vi "channels_get.vi"(8 "error in (no error)":errorcluster, 11 "OSA300 in":refnum<class "OSA300.lvclass">) -> (0 "error out":errorcluster, 1 "channel properties":T1(array[cluster]), 2 "channels nr":i32, 3 "OSA300 out":refnum<class "OSA300.lvclass">)   [LabVIEW 2010, in "OSA300.lvclass"]
uses:
  OSA300.lvclass
  _OSAchannel_class/OSAchannel.lvclass
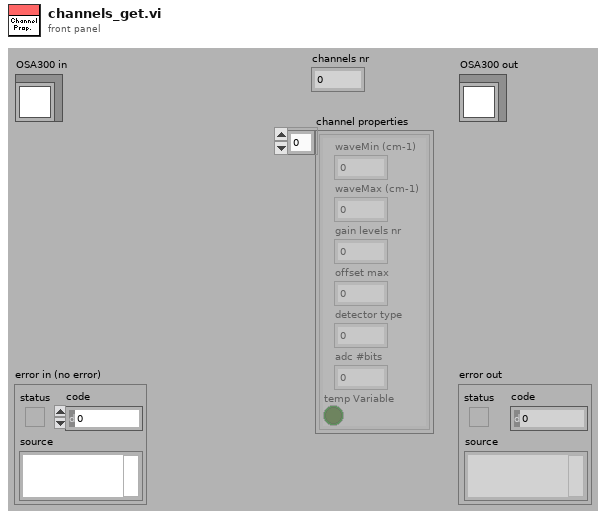
[diagram p1: front panel]
types:
  T1 = cluster{"waveMin (cm-1)":sgl, "waveMax (cm-1)":sgl, "gain levels nr":u16, "offset max":u16, "detector type":i32, "adc #bits":dbl, "temp Variable":bool}[]
  T2 = typedef "OSA20X_misc.lvlib/amplifier_sort.ctl" = enum16{"amp_unknown", "amp_se_8", "amp_se_12_lg", "amp_se_12", "amp_se_16", "amp_diff_8", "amp_diff_12_lg", "amp_diff_12_ir", "amp_diff_16", "amp_other", "amp_other_2"}
  T3 = typedef "OSA20X_misc.lvlib/detector_sort.ctl" = enum16{"unknown", "Silicon", "Silicon PIN", "Silicon MPPC", "InGaAs", "InGaAs ext low", "InGaAs ext high", "InAs", "InAsSb", "InSb", "MCT", "other", "other2", "other3"}
  T4 = typedef "OSA20X_misc.lvlib/interferogram_smoothing.ctl" = enum16{"NONE", "BINOMIAL", "SAVITSKY_GOLAY", "FOURIER", "MOVING_AVERAGE", "GAUSSIAN"}
  T5 = typedef "OSA20X_misc.lvlib/PDTemperatureMode.ctl" = enum16{"cool: better sensitivity/noise floor", "warm: extended wl range"}
  T6 = cluster{"waveMin (cm-1)":sgl, "waveMax (cm-1)":sgl, "gainOffset_auto":bool, "gain":i32, "gain levels nr":u16, "offset":i32, "offset max":u16, "damper available":bool, "damper active":bool, "amplifier sort":T2, "detector sort":T3, "channelIdx global":u16, "spectrIdx":u16, "waveMeter on":bool, "ref gainLevels rel.":refnum<data-value>, "intfgrm_smooth_width":u16, "intfgrm_smooth_nrOfPasses":u16, "intfgrm_smooth":T4, "adc #bits":u16, "temp Variable":bool, "spectr_smooth":T4, "spectr_smooth_width":u16, "spectr_smooth_nrOfPasses":u16, "PD sensitivity mode":T5, "damper auto":bool}
  T7 = cluster{"waveMin (cm-1)":sgl, "waveMax (cm-1)":sgl, "gain levels nr":u16, "offset max":u16, "detector sort":T3, "adc #bits":u16, "temp Variable":bool}
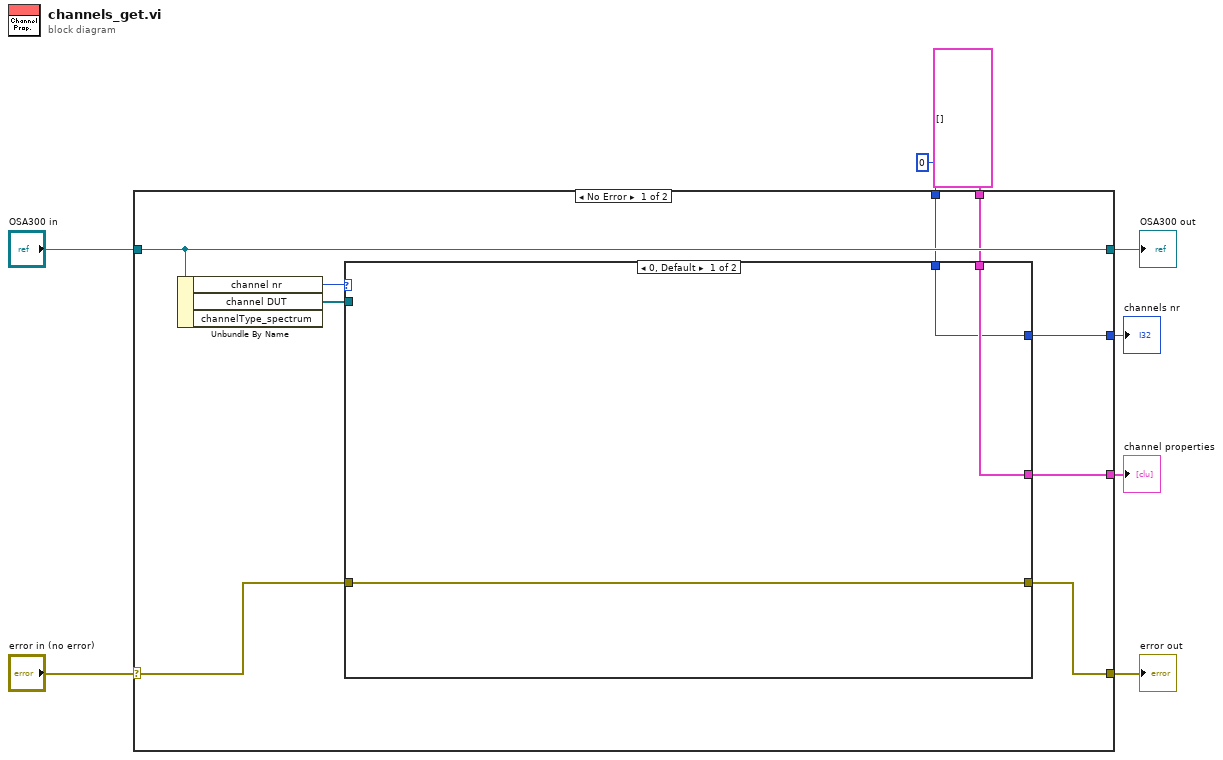
[diagram p0: block diagram]
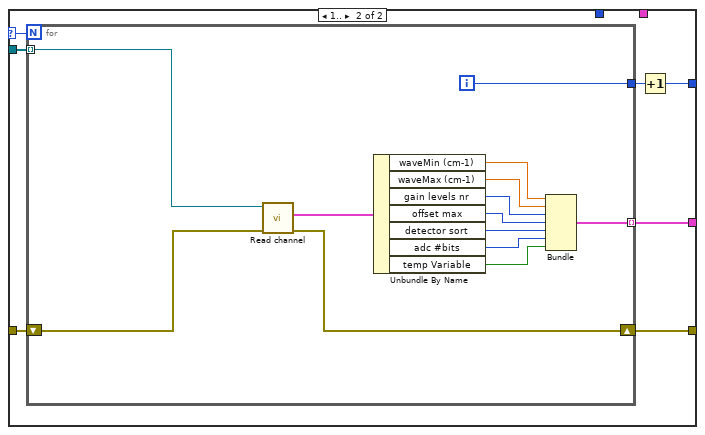
[diagram p2: hidden frame]
diagram:
  n1 = case shown="No Error" "error in (no error)" {
    selector: "error in (no error)" -> [w15 w44]
    tunnel: [w11 w44] -> w7
    tunnel: [w16 w43] -> w5
    tunnel: "OSA300 in" -> [w16 w43]
    tunnel: [w13 w42] -> w4
    tunnel: [w12 w41] -> w3
    tunnel: 0 -> [w9 w42]
    tunnel: T1 [] -> [w10 w41]
    frame No Error {
      n2 = Unbundle By Name(w16) -> ("channel nr"=w14:i32, "channel DUT"=w17:refnum<class "OSAchannel.lvclass">[])  [unwired: 1 out]
      n3 = case shown="0, Default" w14 {
        selector: w14 -> [_ w25]
        tunnel: w17 -> [_ w27]
        tunnel: w15 -> [w20 w26]
        tunnel: [w18 w23] -> w13
        tunnel: [w19 w22] -> w12
        tunnel: [w20 w21] -> w11
        tunnel: w10 -> [w19 _]
        tunnel: w9 -> [w18 _]
        frame 0, Default {
        }
        frame 1.. {
          n4 = for {
            N: w25 -> [_]
            tunnel: w27 -> [w40] mode=indexing
            shift-right: [w28] -> w21
            shift-left: w26 -> [w39]
            tunnel: [w37] -> w24
            tunnel: [w29] -> w22 mode=indexing
            i -> [w37]
            n5 = call "Read channel.vi"("error in (no error)"=w39, "OSAchannel in"=w40) -> ("error out"=w28:errorcluster, "channel"=w38:T6)  [unwired: 7 in, 1 out]
            n6 = Unbundle By Name(w38) -> ("waveMin (cm-1)"=w36:sgl, "waveMax (cm-1)"=w35:sgl, "gain levels nr"=w34:u16, "offset max"=w33:u16, "detector sort"=w32:T3, "adc #bits"=w31:u16, "temp Variable"=w30:bool)
            n7 = Bundle("waveMin (cm-1)"=w36, "waveMax (cm-1)"=w35, "gain levels nr"=w34, "offset max"=w33, "detector sort"=w32, "adc #bits"=w31, "temp Variable"=w30) -> (w29:T7)  [unwired: 1 in]
          }
          n8 = Increment(x=w24) -> (x+1=w23:i32)
        }
      }
    }
    frame Error {
    }
  }
  "error out" <- w7
  "OSA300 out" <- w5
  "channels nr" <- w4
  "channel properties" <- w3
